vi "Read IQ Recorder Measurement IQ Amplitudes.vi"(8 "error in (no error)":errorcluster, 10 "Instance (1)":i32=1 format="%.0g", 11 "VISA resource name":refnum<visa-resource-name>) -> (0 "error out":errorcluster, 1 "I Amplitudes":dbl[](array[numeric]) format="%.2p", 2 "Reliability":i32, 3 "VISA resource name out":refnum<visa-resource-name>, 4 "Q Amplitudes":dbl[](array[numeric]) format="%.2p")   [LabVIEW 2015, in "Rohde&Schwarz CMXP GPRF.lvlib"]
doc: "Starts a new single shot measurement and returns the I and Q amplitudes.\n\nAttribute:\nRSCMXPGPRF_ATTR_READ_IQ_RECORDER_MEASUREMENT_IQ_AMPLITUDES\n\nRemote-control command:\nREAD:GPRF:MEAS<i>:IQRecorder?"
uses:
  <instrlib>/Rohde&Schwarz CMXP GPRF/Rohde&Schwarz CMXP GPRF.lvlib
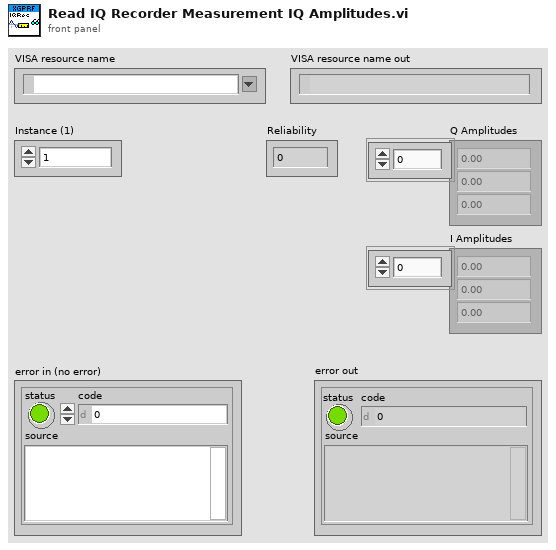
[diagram p1: front panel]
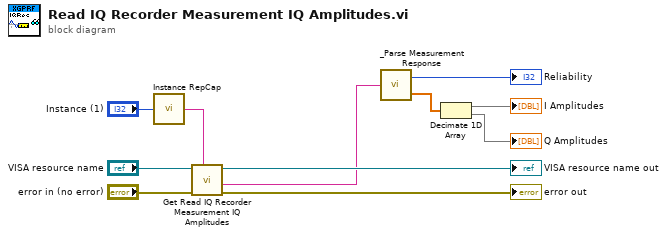
[diagram p0: block diagram]
diagram:
  n1 = call <instrlib>:"Instance RepCap.vi"("instance  in"="Instance (1)") -> ("instance out"=w6:string)
  n2 = call "Get Read IQ Recorder Measurement IQ Amplitudes"("Repeated Capabilities"=w6, "error in (no error)"="error in (no error)", "instrument handle"="VISA resource name") -> ("error out"=→"error out":errorcluster, "Read IQ Recorder Measurement IQ Amplitudes"=w1:string, "instrument handle out"=→"VISA resource name out":refnum<visa-resource-name>)  [unwired: 6 in]
  n3 = call <instrlib>:"_Parse Measurement Response.vi"("String In"=w1) -> ("Reliability"=→"Reliability":i32, "Data"=w3:dbl[])
  n4 = Decimate 1D Array(w3) -> (→"I Amplitudes":dbl[], →"Q Amplitudes":dbl[])
